vi "DirettoreStop.vi"(11 "FPGAReference":refnum<k20>) -> (0 "ErrorOut":errorcluster)   [LabVIEW 2012]
uses:
  <vilib>/FPGAPlugInAG/Dynamic/niLvFpga_Abort_Dynamic.vi
  <vilib>/rvi/interface/nirviMethod/nirviMethod.xnode
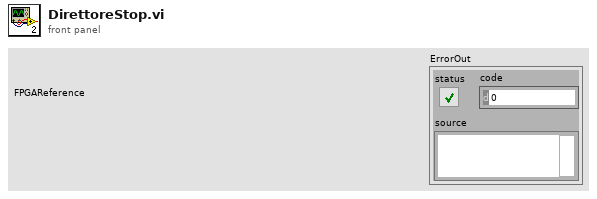
[diagram p1: front panel]
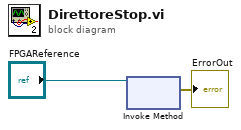
[diagram p0: block diagram]
diagram:
  n1 = xnode "Invoke Method"("FPGA VI Reference In"="FPGAReference") -> ("error out"=→"ErrorOut":errorcluster)  [unwired: 1 in, 1 out]
